vi "Data-to-PC.vi"() -> (2 "Data":dbl[][](array[numeric]))   [LabVIEW 2018]
uses:
  <vilib>/Utility/file.llb/Write Delimited Spreadsheet (DBL).vi
panel:
  out "State":enum16{"Initialize", "Wait", "Save", "Stop"}(ring)
  in  "Filename":string
  in  "Stop":bool
  in  "Start":bool
  out "path":path
  out "Time":dbl[](array[numeric])
  out "EEG":dbl[](array[numeric])
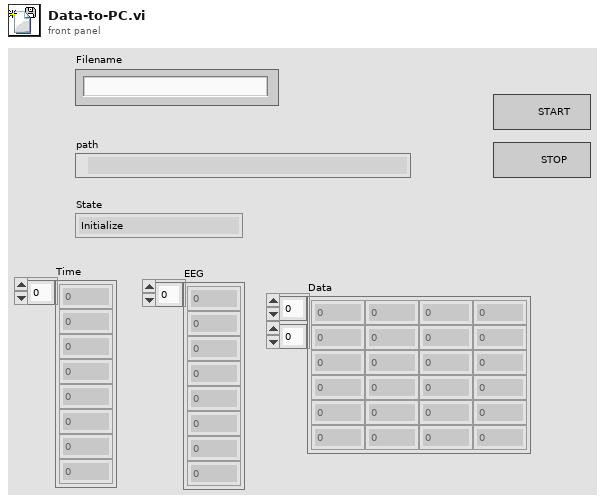
[diagram p1: front panel]
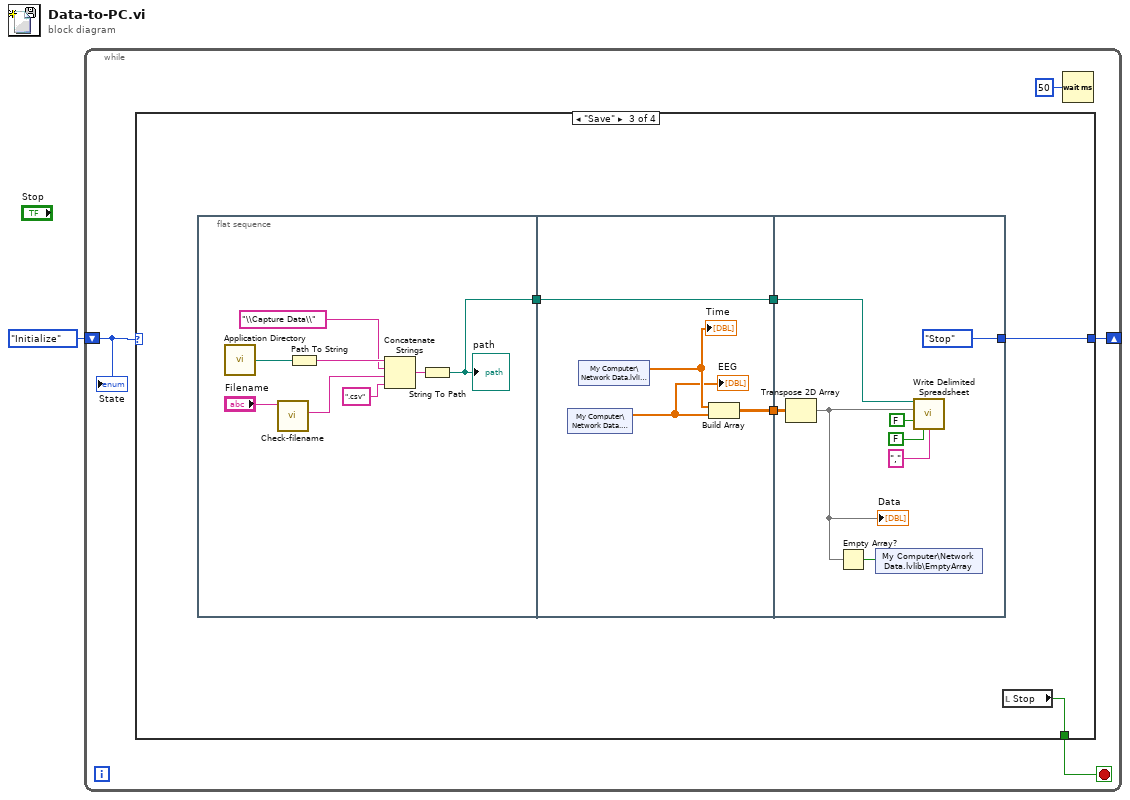
[diagram p0: block diagram]
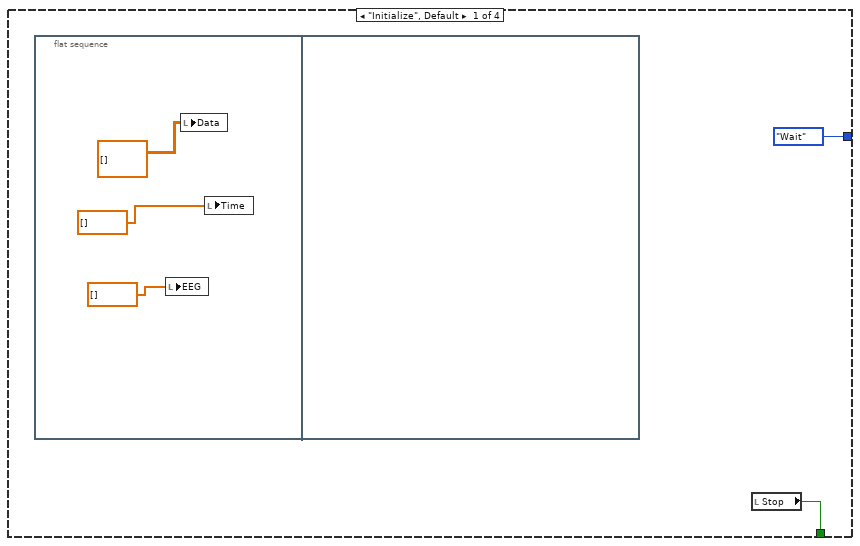
[diagram p2: hidden frame]
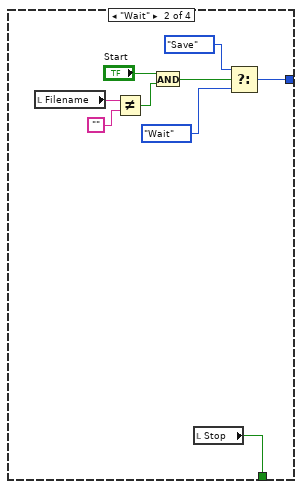
[diagram p3: hidden frame]
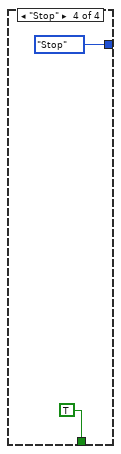
[diagram p4: hidden frame]
diagram:
  n1 = while {
    shift-right: [w3] -> _
    shift-left: enum16{"Initialize", "Wait", "Save", "Stop"}."Initialize" -> [w5]
    stop <- w4 stop-if-true
    n2 = case shown="\"Save\"" w5 {
      tunnel: [w6 w19 w20 TRUE] -> w4
      tunnel: [enum16{"Initialize", "Wait", "Save", "Stop"}."Wait" w11 w21 enum16{"Initialize", "Wait", "Save", "Stop"}."Stop"] -> w3
      frame "Initialize", Default {
        n3 = flat-sequence {
          frame #0 {
            n4 = local write "EEG"(dbl[] []) -> ()
            n5 = local write "Data"(dbl[][] []) -> ()
            n6 = local write "Time"(dbl[] []) -> ()
          }
          frame #1 {
          }
        }
        n7 = local read "Stop"() -> (w6:bool)
      }
      frame "Wait" {
        n8 = local read "Filename"() -> (w17:string)
        n9 = Not Equal?(x=w17, y="") -> (x != y?=w15:bool)
        n10 = And(x="Start", y=w15) -> (x .and. y?=w14:bool)
        n11 = local read "Stop"() -> (w19:bool)
        n12 = Select(t=enum16{"Initialize", "Wait", "Save", "Stop"}."Save", s=w14, f=enum16{"Initialize", "Wait", "Save", "Stop"}."Wait") -> (s? t:f=w11:enum16{"Initialize", "Wait", "Save", "Stop"})
      }
      frame "Save" {
        n13 = flat-sequence {
          tunnel: [w27] -> w24
          tunnel: [w35] -> w23
          tunnel: [w33] -> w22
          tunnel: w24 -> [w33]
          tunnel: w23 -> [w41]
          tunnel: w22 -> [w40]
          tunnel: [enum16{"Initialize", "Wait", "Save", "Stop"}."Stop"] -> w21
          frame #0 {
            n14 = call <vilib>:"Application Directory.vi"() -> ("Application Directory"=w31:path)
            n15 = call "Check-filename.vi"("Filename"="Filename") -> ("Filename (Evaluated)"=w26:string)  [unwired: 10 in]
            n16 = Path To String(path=w31) -> (string=w30:string)
            n17 = Concatenate Strings(w30, "\\Capture Data\\" ("string"), w26, ".csv" ("string")) -> (w32:string)
            n18 = String To Path(string=w32) -> (path=w27:path)
            "path" <- w27
          }
          frame #1 {
            n19 = shared-variable "My Computer\\Network Data.lvlib\\EEG"() -> (w34:dbl[])  [unwired: 1 in, 1 out]
            "EEG" <- w34
            n20 = shared-variable "My Computer\\Network Data.lvlib\\Time"() -> (w36:dbl[])  [unwired: 1 in, 1 out]
            "Time" <- w36
            n21 = Build Array(w36, w34) -> (w35:dbl[][])
          }
          frame #2 {
            n22 = Transpose 2D Array(2D array=w41) -> (transposed array=w37:dbl[][])
            "Data" <- w37
            n23 = Empty Array?(array=w37) -> (empty?=w38:bool)
            n24 = shared-variable "My Computer\\Network Data.lvlib\\EmptyArray"(w38) -> ()  [unwired: 1 in, 1 out]
            n25 = call-poly <vilib>:"Write Delimited Spreadsheet.vi"("file path (dialog if empty)"=w40, "2D data"=w37, "append to file? (new file:F)"=FALSE, "transpose? (no:F)"=FALSE, "delimiter (\\t)"="," ("delimiter (\\t)")) -> ()  [unwired: 9 in, 2 out]
          }
        }
        n26 = local read "Stop"() -> (w20:bool)
      }
      frame "Stop" {
      }
    }
    n27 = Wait (ms)(milliseconds to wait=u32 50) -> ()  [unwired: 1 out]
    "State" <- w5
  }
